vi "Plugin -Short Offset.vi"(11 "Message Queues in":T2) -> ()   [LabVIEW 2019]
uses:
  support/Copy of Message Queue/All Message Queues.ctl
  support/Copy of Message Queue/Message Cluster.ctl
  controls/WhieBackgroundHistogram.ctl
  support/Message Queue/Message Queue.lvlib
  support/Copy of Message Queue/Copy of Message Queue.lvlib
panel:
  in  "Stop":bool
  out "Time vs. Offset/Cor Offset":dbl(graph)
  out "Histogram Graph":T1
  out "T12":dbl(slide) scale=0.0..30.0
  out "T11":dbl(slide) scale=0.0..30.0
  out "T10":dbl(slide) scale=0.0..30.0
  out "T9":dbl(slide) scale=0.0..30.0
  out "T8":dbl(slide) scale=0.0..30.0
  out "T7":dbl(slide) scale=0.0..30.0
  out "T6":dbl(slide) scale=0.0..30.0
  out "T5":dbl(slide) scale=0.0..30.0
  out "T4":dbl(slide) scale=0.0..30.0
  out "T3":dbl(slide) scale=0.0..30.0
  out "T2":dbl(slide) scale=0.0..30.0
  out "T1":dbl(slide) scale=0.0..30.0
  out "Ring Time":waveform(dbl)[](graph)
  out "Aquatrak RS232 Output":string
  in  "error in":errorcluster
  out "error out":errorcluster
  # "Calulating Short Offset"
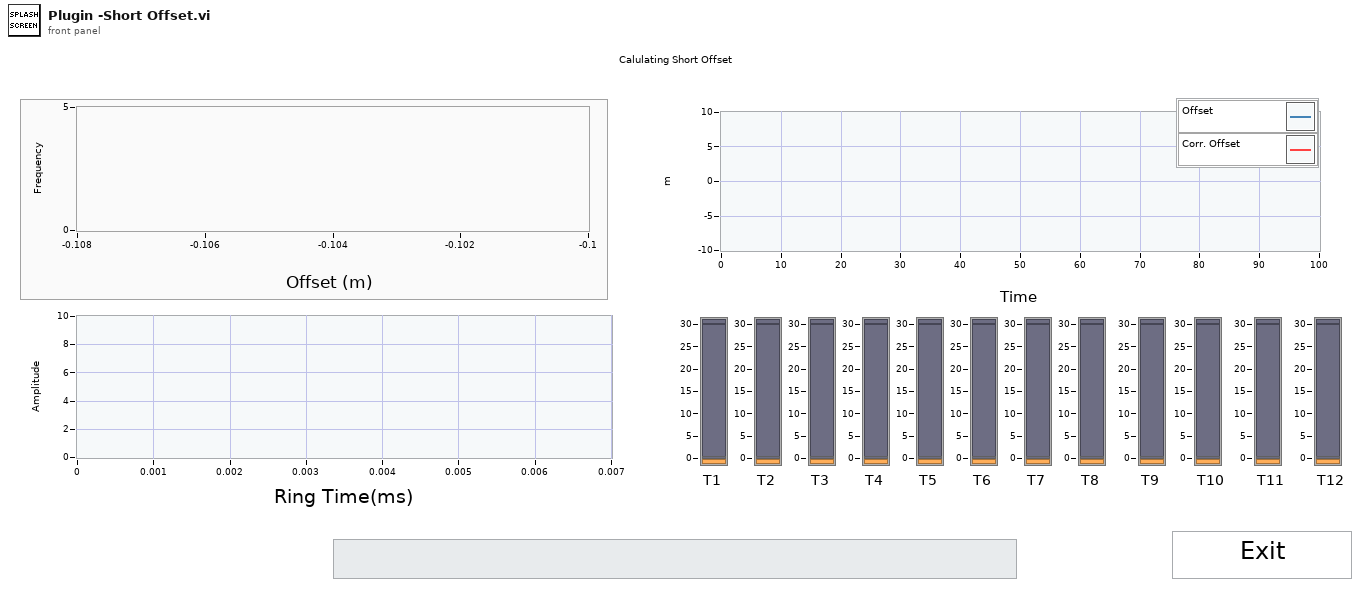
[diagram p1: front panel]
types:
  T1 = typedef "WhieBackgroundHistogram.ctl" = cluster{"X Values":dbl[], "Histogram: h(x)":i32[]}
  T2 = typedef "Copy of Message Queue.lvlib/All Message Queues.ctl" = cluster{"UI":refnum<queue>, "Acquisition":refnum<queue>, "Logging":refnum<queue>, "Analyze":refnum<queue>}
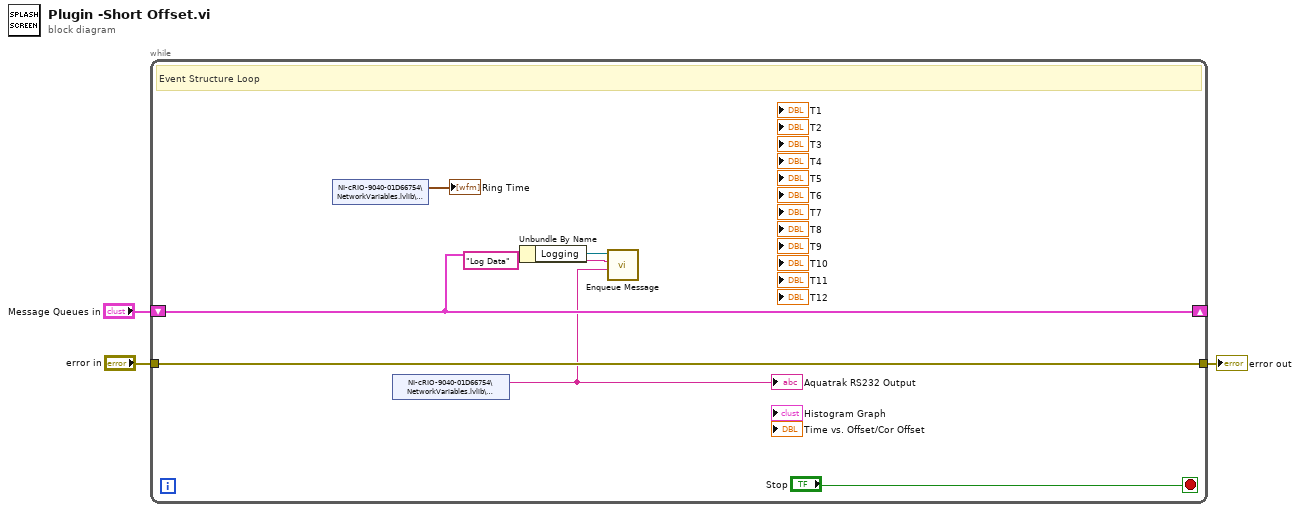
[diagram p0: block diagram]
diagram:
  n1 = while {
    shift-right: [w5] -> _
    shift-left: "Message Queues in" -> [w5]
    tunnel: [w10] -> w2
    tunnel: "error in" -> [w10]
    stop <- "Stop" stop-if-true
    # "Event Structure Loop"
    n2 = shared-variable "NI-cRIO-9040-01D66754\\NetworkVariables.lvlib\\RingTime"() -> (→"Ring Time":waveform(dbl)[])  [unwired: 1 in, 1 out]
    n3 = shared-variable "NI-cRIO-9040-01D66754\\NetworkVariables.lvlib\\AquatrakData"() -> (w4:string)  [unwired: 1 in, 1 out]
    "Aquatrak RS232 Output" <- w4
    n4 = Unbundle By Name(w5) -> ("Logging"=w6:refnum<queue>)
    n5 = call "Enqueue Message.vi"("Message Data"=w4, "Message"="Log Data", "Message Queue"=w6) -> ()  [unwired: 7 in, 2 out]
  }
  "error out" <- w2
